vi "Meas Result Generate TWM Correction - Parametric Uncertainty Generate.vi"(7 "unc params":T1, 8 "error in (no error)":errorcluster, 9 "minor":dbl, 10 "major":dbl, 11 "f [Hz]":dbl) -> (0 "error out":errorcluster, 1 "u(mnr)":dbl, 2 "u(mjr)":dbl, 4 "u(mjr) [%]":dbl, 6 "u(mnr) [%]":dbl)   [LabVIEW 2020]
doc: "Generates parametric uncertainty for given values."
uses:
  Meas Results TWM Correction Uncertainty Parametric Generator Ctrls.ctl
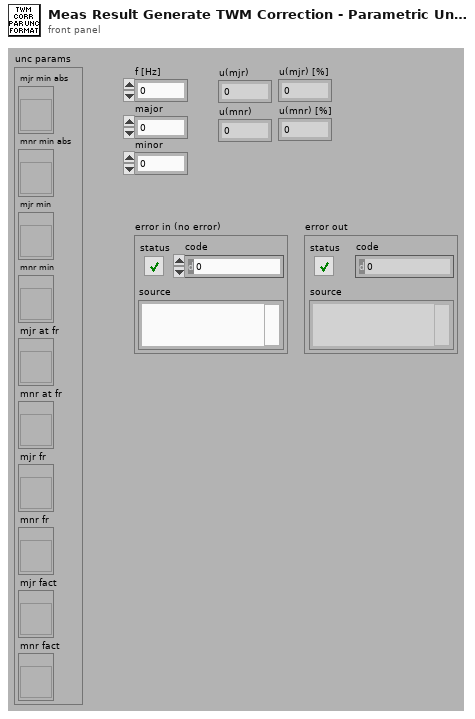
[diagram p1: front panel]
types:
  T1 = typedef "Meas Results TWM Correction Uncertainty Parametric Generator Ctrls.ctl" = cluster{"mjr min abs":refnum<vi>, "mnr min abs":refnum<vi>, "mjr min":refnum<vi>, "mnr min":refnum<vi>, "mjr at fr":refnum<vi>, "mnr at fr":refnum<vi>, "mjr fr":refnum<vi>, "mnr fr":refnum<vi>, "mjr fact":refnum<vi>, "mnr fact":refnum<vi>}
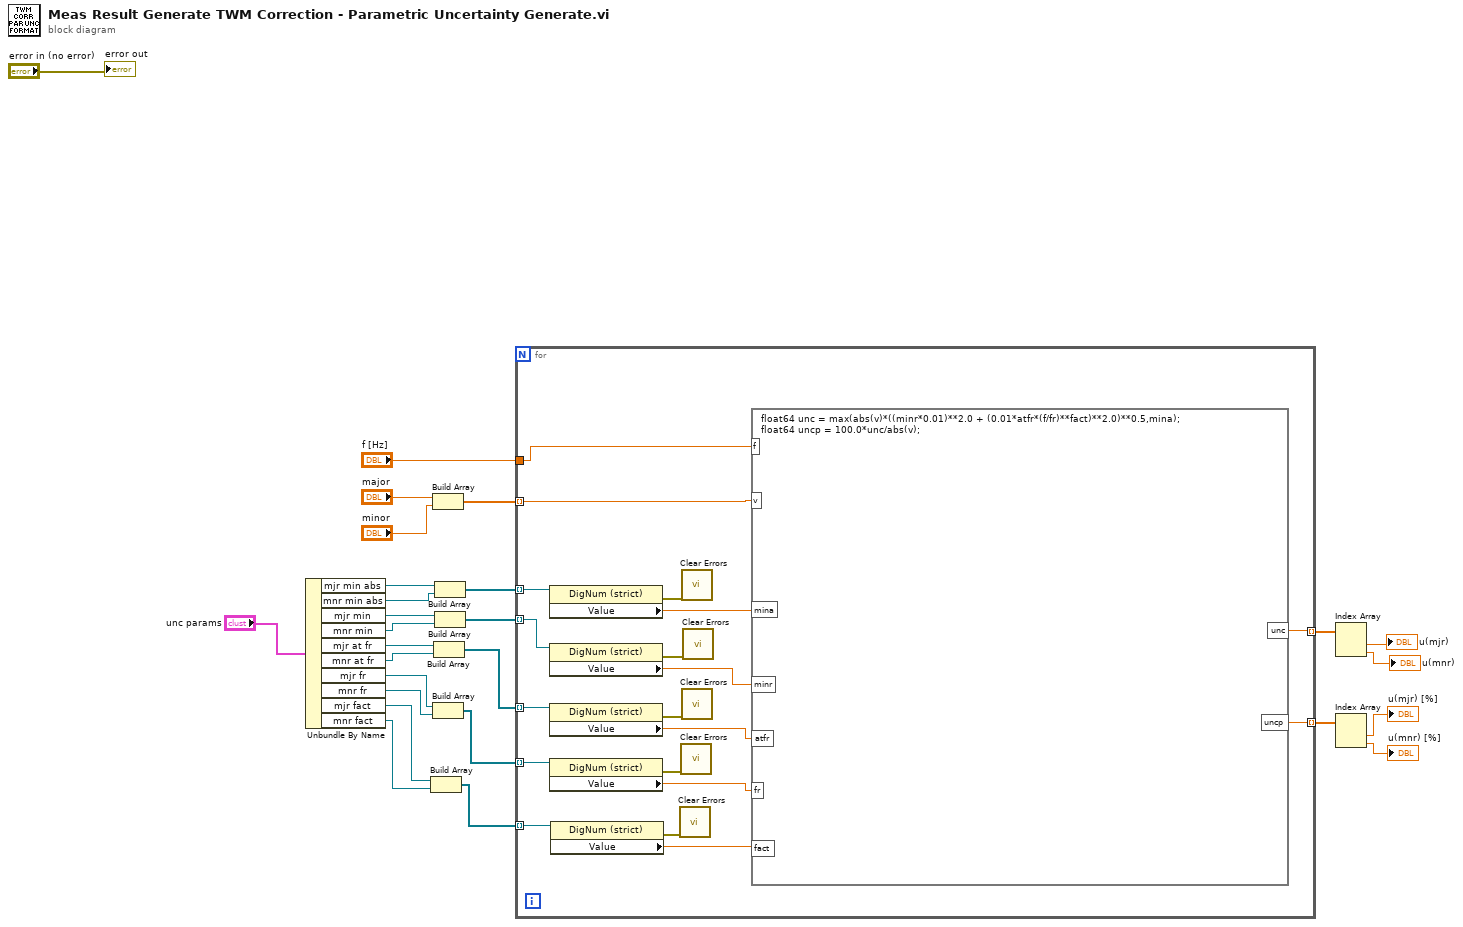
[diagram p0: block diagram]
diagram:
  n1 = Unbundle By Name("unc params") -> ("mjr min abs"=w26:refnum<vi>, "mnr min abs"=w25:refnum<vi>, "mjr min"=w23:refnum<vi>, "mnr min"=w22:refnum<vi>, "mjr at fr"=w20:refnum<vi>, "mnr at fr"=w19:refnum<vi>, "mjr fr"=w17:refnum<vi>, "mnr fr"=w16:refnum<vi>, "mjr fact"=w14:refnum<vi>, "mnr fact"=w13:refnum<vi>)
  n2 = Build Array(w14, w13) -> (w12:refnum<vi>[])
  n3 = Build Array("major", "minor") -> (w7:dbl[])
  n4 = Build Array(w17, w16) -> (w15:refnum<vi>[])
  n5 = Build Array(w20, w19) -> (w18:refnum<vi>[])
  n6 = Build Array(w26, w25) -> (w24:refnum<vi>[])
  n7 = Build Array(w23, w22) -> (w21:refnum<vi>[])
  n8 = for {
    tunnel: w24 -> [w46] mode=indexing
    tunnel: w21 -> [w45] mode=indexing
    tunnel: w18 -> [w44] mode=indexing
    tunnel: w15 -> [w43] mode=indexing
    tunnel: w12 -> [w42] mode=indexing
    tunnel: "f [Hz]" -> [w36]
    tunnel: w7 -> [w35] mode=indexing
    tunnel: [w29] -> w6 mode=indexing
    tunnel: [w28] -> w3 mode=indexing
    n9 = property class="DigNum (strict)"(reference=w46) -> (error out=w41:errorcluster, "Value"=w34:dbl)  [unwired: 1 in, 1 out]
    n10 = property class="DigNum (strict)"(reference=w45) -> (error out=w40:errorcluster, "Value"=w33:dbl)  [unwired: 1 in, 1 out]
    n11 = property class="DigNum (strict)"(reference=w44) -> (error out=w39:errorcluster, "Value"=w32:dbl)  [unwired: 1 in, 1 out]
    n12 = property class="DigNum (strict)"(reference=w43) -> (error out=w38:errorcluster, "Value"=w31:dbl)  [unwired: 1 in, 1 out]
    n13 = property class="DigNum (strict)"(reference=w42) -> (error out=w37:errorcluster, "Value"=w30:dbl)  [unwired: 1 in, 1 out]
    n14 = call <vilib>:"Clear Errors.vi"("error in (no error)"=w37) -> ()  [unwired: 5 in, 2 out]
    n15 = call <vilib>:"Clear Errors.vi"("error in (no error)"=w38) -> ()  [unwired: 5 in, 2 out]
    n16 = call <vilib>:"Clear Errors.vi"("error in (no error)"=w41) -> ()  [unwired: 5 in, 2 out]
    n17 = call <vilib>:"Clear Errors.vi"("error in (no error)"=w39) -> ()  [unwired: 5 in, 2 out]
    n18 = call <vilib>:"Clear Errors.vi"("error in (no error)"=w40) -> ()  [unwired: 5 in, 2 out]
    n19 = formula code="float64 unc = max(abs(v)*((minr*0.01)**2.0 + (0.01*atfr*(f/fr)**fact)**2.0)**0.5,mina);\nfloat64 uncp = 100.0*unc/abs(v);"("f"=w36, "v"=w35, "mina"=w34, "minr"=w33, "atfr"=w32, "fr"=w31, "fact"=w30) -> ("unc"=w29:dbl, "uncp"=w28:dbl)
  }
  n20 = Index Array(array=w6) -> (element #1=→"u(mjr)":dbl, element #2=→"u(mnr)":dbl)  [unwired: 2 in]
  n21 = Index Array(array=w3) -> (element #1=→"u(mjr) [%]":dbl, element #2=→"u(mnr) [%]":dbl)  [unwired: 2 in]
  "error out" <- "error in (no error)"
